vi "Test if vis with prefix can be found.vi"(8 "error in":errorcluster, 11 "TestCase in":refnum<class "Tree Selection.lvclass">) -> (0 "error out":errorcluster, 3 "TestCase out":refnum<class "Tree Selection.lvclass">)   [LabVIEW 2019, in "Tree Selection.lvclass"]
uses:
  Tree Selection.lvclass
  Panther Dashboard Project/Panther Dashboard/Panther Dashboard/Panther Dashboard.lvlib
  Test Library/Test Library.lvlib
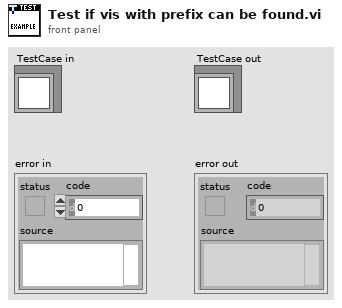
[diagram p1: front panel]
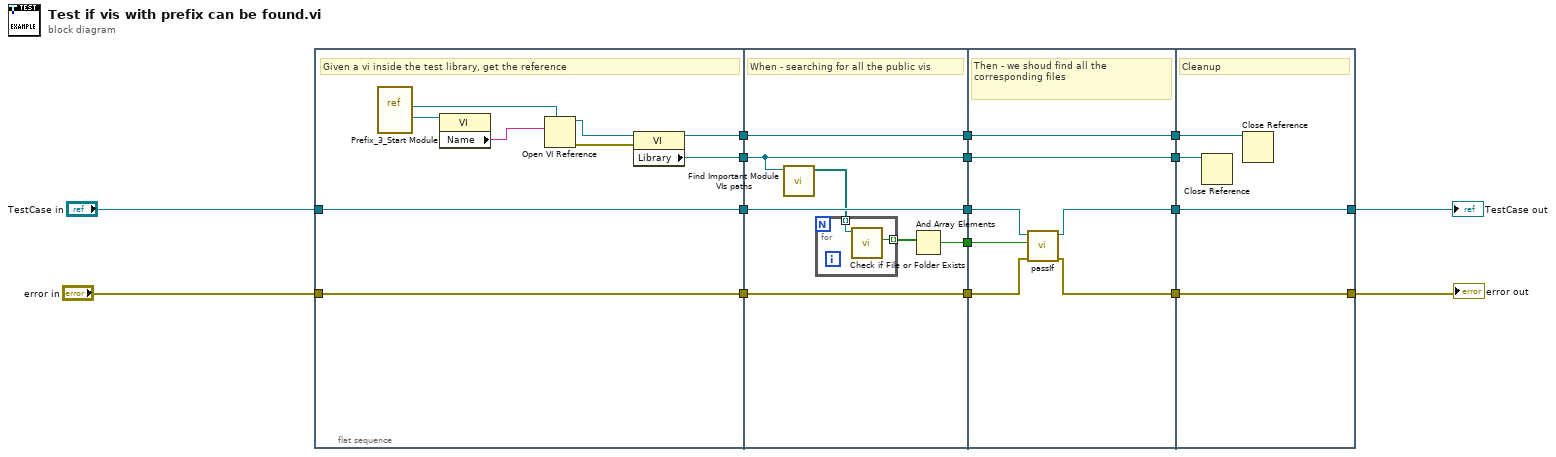
[diagram p0: block diagram]
diagram:
  n1 = flat-sequence {
    tunnel: "error in" -> [w25]
    tunnel: "TestCase in" -> [w23]
    tunnel: [w23] -> w12
    tunnel: [w25] -> w17
    tunnel: [w21] -> w6
    tunnel: [w20] -> w5
    tunnel: [w31] -> w11
    tunnel: [w32] -> w16
    tunnel: w12 -> [w31]
    tunnel: w17 -> [w32]
    tunnel: [w28] -> w7
    tunnel: w6 -> [w26]
    tunnel: w5 -> [w27]
    tunnel: [w27] -> w4
    tunnel: [w26] -> w2
    tunnel: [w38] -> w10
    tunnel: [w40] -> w15
    tunnel: w11 -> [w39]
    tunnel: w16 -> [w41]
    tunnel: w7 -> [w37]
    tunnel: w4 -> [w36]
    tunnel: [w36] -> w3
    tunnel: w2 -> [w35]
    tunnel: [w35] -> w1
    tunnel: [w45] -> w13
    tunnel: [w44] -> w8
    tunnel: w10 -> [w44]
    tunnel: w15 -> [w45]
    tunnel: w3 -> [w43]
    tunnel: w1 -> [w42]
    frame #0 {
      # "Given a vi inside the test library, get the reference"
      n2 = vi-ref "Prefix_3_Start Module.vi"() -> (w18:refnum<vi>)
      n3 = property class="VI"(reference=w18) -> ("Name"=w19:string)  [unwired: 1 in, 2 out]
      n4 = Open VI Reference(type specifier VI Refnum (for type only)=w18, vi path=w19) -> (vi reference=w22:refnum<vi>, error out=w24:errorcluster)  [unwired: 4 in]
      n5 = property class="VI"(reference=w22, error in=w24) -> (reference out=w20:refnum<vi>, "Library"=w21:refnum<vi>)  [unwired: 1 out]
    }
    frame #1 {
      # "When - searching for all the public vis"
      n6 = call "Find Important Module VIs paths.vi"("Library in"=w26) -> ("Public API VIs Paths"=w30:path[])  [unwired: 10 in]
      n7 = for {
        tunnel: w30 -> [w34] mode=indexing
        tunnel: [w33] -> w29 mode=indexing
        n8 = call <vilib>:"Check if File or Folder Exists.vi"("path"=w34) -> ("file or folder exists?"=w33:bool)  [unwired: 8 in, 2 out]
      }
      n9 = And Array Elements(Boolean array=w29) -> (logical AND=w28:bool)
    }
    frame #2 {
      # "Then - we shoud find all the corresponding files"
      n10 = call-dynamic "passIf.vi"("error in (no error)"=w41, "pass"=w37, "TestCase in"=w39) -> ("error out"=w40:errorcluster, "TestCase out"=w38:refnum<class "Tree Selection.lvclass">)  [unwired: 7 in]
    }
    frame #3 {
      # "Cleanup"
      n11 = Close Reference(reference=w42) -> ()  [unwired: 1 in, 1 out]
      n12 = Close Reference(reference=w43) -> ()  [unwired: 1 in, 1 out]
    }
  }
  "error out" <- w13
  "TestCase out" <- w8
